vi "Verify User Access.vi"(8 "error in (no error)":errorcluster, 9 "Password Input":string, 10 "Username":string, 11 "UserPwd DB in":refnum<class "UserPwd DB.lvclass">) -> (0 "error out":errorcluster, 1 "Access":T1, 2 "Valid":bool, 3 "UserPwd DB out":refnum<class "UserPwd DB.lvclass">, 4 "Permission":u32)   [LabVIEW 2016, in "UserPwd DB.lvlib" / "UserPwd DB.lvclass"]
uses:
  <userlib>/Common Components/UserPwd DB/UserPwd DB/UserPwd DB.lvclass
  <userlib>/Common Components/UserPwd DB/UserPwd DB/Access Level.ctl
  <userlib>/Common Components/UserPwd DB/UserPwd DB/UserPwd DB.lvclass/UserPwd DB.ctl
  <userlib>/Common Components/UserPwd DB/UserPwd DB/Data saved.ctl
  <vilib>/addons/_JKI.lib/Serialization/JSON/JKI JSON Serialization.lvlib
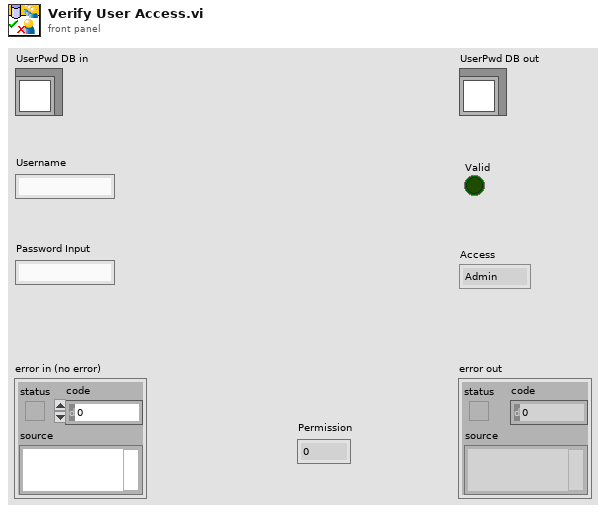
[diagram p1: front panel]
types:
  T1 = typedef "UserPwd DB.lvlib/UserPwd DB.lvclass/Access Level.ctl" = enum16{"Admin", "User lv1", "User lv2", "User lv3", "User lv4", "User lv5", "User lv6", "User lv7", "User lv8", "User lv9", "Guest"}
  T2 = typedef "UserPwd DB.lvlib/UserPwd DB.lvclass/Data saved.ctl" = cluster{"Encrypted Password":string, "Access":T1, "Permission":u32}
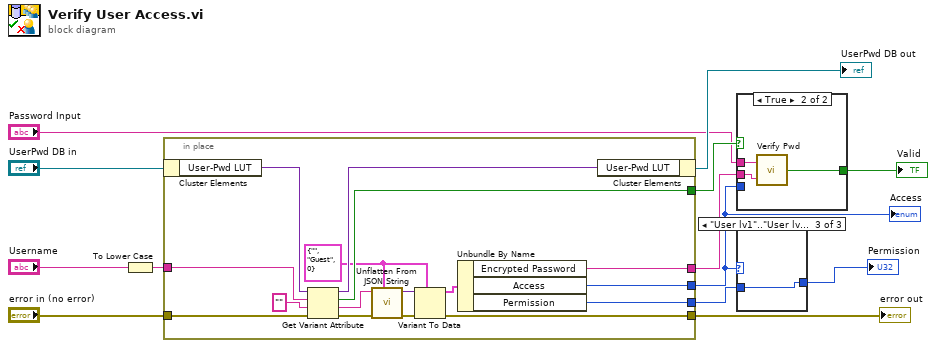
[diagram p0: block diagram]
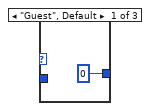
[diagram p2: hidden frame]
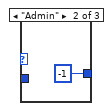
[diagram p3: hidden frame]
diagram:
  n1 = To Lower Case(string="Username") -> (all lower case string=w5:string)
  n2 = in-place {
    in-place-border: w5 -> [w27]
    in-place-border: "error in (no error)" -> [w26]
    in-place-border: [w18] -> w9
    in-place-border: [w24] -> w3
    in-place-border: [w23] -> w8
    in-place-border: [w22] -> w6
    in-place-border: [w14] -> w1
    w17 = T2 {"Encrypted Password"="", "Access"=enum."Guest", "Permission"=0} ("Data")
    n3 = in-place-cluster #1("UserPwd DB in") -> ("User-Pwd LUT"=w29:variant)
    n4 = Get Variant Attribute(Variant=w29, name=w27, default value (empty Variant)="" ("Password"), error in=w26) -> (duplicate Variant=w28:variant, found=w23:bool, value=w19:string, error out=w25:errorcluster)
    n5 = call <vilib>:"Unflatten From JSON String.vi"("Type and Defaults"=w17, "error in (no error)"=w25, "JSON String"=w19) -> ("error out"=w20:errorcluster, "Variant"=w15:variant)  [unwired: 7 in]
    n6 = Variant To Data(error in=w20, type=w17, Variant=w15) -> (data=w16:T2, error out=w18:errorcluster)
    n7 = Unbundle By Name(w16) -> ("Encrypted Password"=w22:string, "Access"=w24:T1, "Permission"=w14:u32)
    n8 = in-place-cluster #1("User-Pwd LUT"=w28) -> (→"UserPwd DB out":refnum<class "UserPwd DB.lvclass">)
  }
  "error out" <- w9
  "Access" <- w3
  n9 = case shown="True" w8 {
    tunnel: "Password Input" -> [_ w31]
    tunnel: w6 -> [_ w32]
    tunnel: [_ w30] -> w4
    tunnel: w3 -> [_ _]
    frame False {
    }
    frame True {
      n10 = call <userlib>:"Verify Pwd.vi"("Encrypted Password"=w32, "Password Input"=w31) -> ("Valid"=w30:bool)
    }
  }
  "Valid" <- w4
  n11 = case shown="\"User lv1\"..\"User lv9\"" w3 {
    tunnel: [u32 0 ("Permission") -1 w35] -> w2
    tunnel: w1 -> [_ _ w35]
    frame "Guest", Default {
    }
    frame "Admin" {
    }
    frame "User lv1".."User lv9" {
    }
  }
  "Permission" <- w2
